vi "Write Nested Actor Type.vi"(10 "Nested Actor Type":T1, 11 "Nested Actor in":refnum<class "Nested Actor.lvclass">) -> (3 "Nested Actor out":refnum<class "Nested Actor.lvclass">)   [LabVIEW 2020, in "Nested Actor.lvlib" / "Nested Actor.lvclass"]
uses:
  Nested Actor.lvclass
  Actor Type.ctl
  Nested Actor.lvclass/Nested Actor.ctl
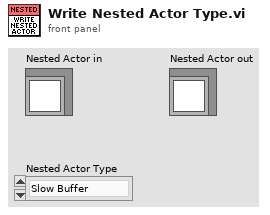
[diagram p1: front panel]
types:
  T1 = typedef "Nested Actor.lvlib/Nested Actor.lvclass/Actor Type.ctl" = enum16{"Slow Buffer", "Fast Buffer"}
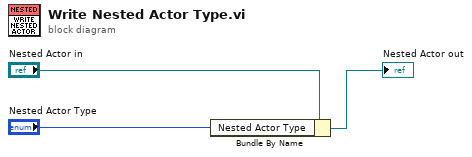
[diagram p0: block diagram]
diagram:
  n1 = Bundle By Name(cluster="Nested Actor in", "Nested Actor Type"="Nested Actor Type") -> (→"Nested Actor out":refnum<class "Nested Actor.lvclass">)
